vi "Close TCP.vi"(8 "error in (no error)":errorcluster, 11 "TCP Comm":T1) -> (0 "error out":errorcluster)   [LabVIEW 2020, in "TinyTCP.lvlib"]
uses:
  TinyTCP.lvlib
  Instance.ctl
  Ref Data.ctl
  State.ctl
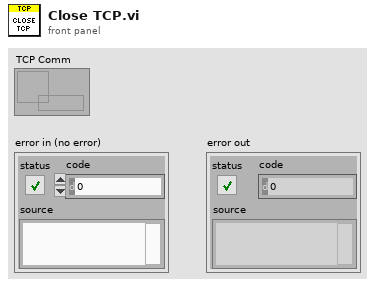
[diagram p1: front panel]
types:
  T1 = typedef "TinyTCP.lvlib/Instance.ctl" = refnum<data-value>
  T2 = typedef "TinyTCP.lvlib/Ref Data.ctl" = cluster{"TCP":refnum<k5>, "State":T3, "Server":bool, "Host":string, "Port":u16, "Listener":refnum<k5>, "Start":bool, "Disconnect":bool, "TCP Valid":bool, "TLS Enabled":bool, "Immutable TLS":refnum<k36>, "Certificate DN":string}
  T3 = typedef "TinyTCP.lvlib/State.ctl" = enum16{"Idle", "Starting", "Connecting", "Connected", "Disconnecting", "Stopped"}
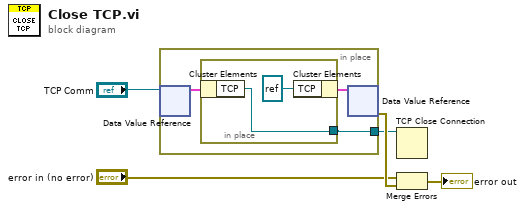
[diagram p0: block diagram]
diagram:
  n1 = in-place {
    in-place-border: [w7] -> w1
    n2 = in-place-dvr #1("TCP Comm") -> (w8:T2)  [unwired: 1 out]
    n3 = in-place {
      in-place-border: [w10] -> w7
      n4 = in-place-cluster #2(w8) -> ("TCP"=w10:refnum<k5>)
      n5 = in-place-cluster #2("TCP"=refnum<k5> refnum) -> (w6:T2)
    }
    n6 = in-place-dvr #1(w6) -> (w5:errorcluster)  [unwired: 1 out]
  }
  n7 = TCP Close Connection(connection ID=w1) -> ()  [unwired: 2 in, 2 out]
  n8 = Merge Errors("error in (no error)", w5) -> (→"error out":errorcluster)
